vi "Initialize.vi"(8 "error in (no error)":errorcluster, 9 "Build Configurations":string[](array[string]), 10 "Preceding Items":refnum<class "Item.lvclass">[](array[class]), 11 "Caraya Item in":refnum<class "Caraya Item.lvclass">) -> (0 "error out":errorcluster, 3 "Item out":refnum<class "Item.lvclass">)   [LabVIEW 2019, in "Caraya Library.lvlib" / "Caraya Item.lvclass"]
uses:
  Caraya Item.lvclass
  C:/Users/pasca/source/repos/mgi-solution-explorer-extensions/libs/Solution.lvlibp/Solution/Item/Item.lvclass
  libs/Solution.lvlibp/Solution/Item/Item.lvclass
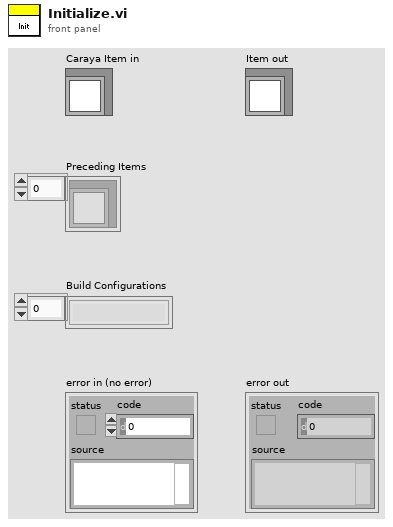
[diagram p1: front panel]
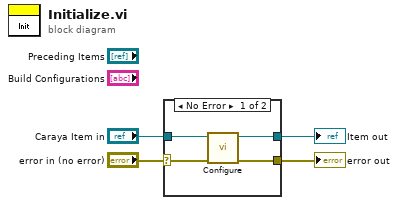
[diagram p0: block diagram]
diagram:
  n1 = case shown="No Error" "error in (no error)" {
    selector: "error in (no error)" -> [w6 w9]
    tunnel: [w8 w9] -> w4
    tunnel: [w7 w10] -> w3
    tunnel: "Caraya Item in" -> [w5 w10]
    frame No Error {
      n2 = call "Configure.vi"("error in (no error)"=w6, "Caraya Item in"=w5) -> ("error out"=w8:errorcluster, "Caraya Item out"=w7:refnum<class "Caraya Item.lvclass">)  [unwired: 8 in]
    }
    frame Error {
    }
  }
  "error out" <- w4
  "Item out" <- w3
